vi "RequestInsertSignals.vi"(5 "Events":T1[](array[typedef]), 11 "error in (no error)":errorcluster) -> (6 "request":string, 15 "error out":errorcluster)   [LabVIEW 2019, in "Logger.lvclass"]
uses:
  Logger.lvclass
  SignalData.ctl
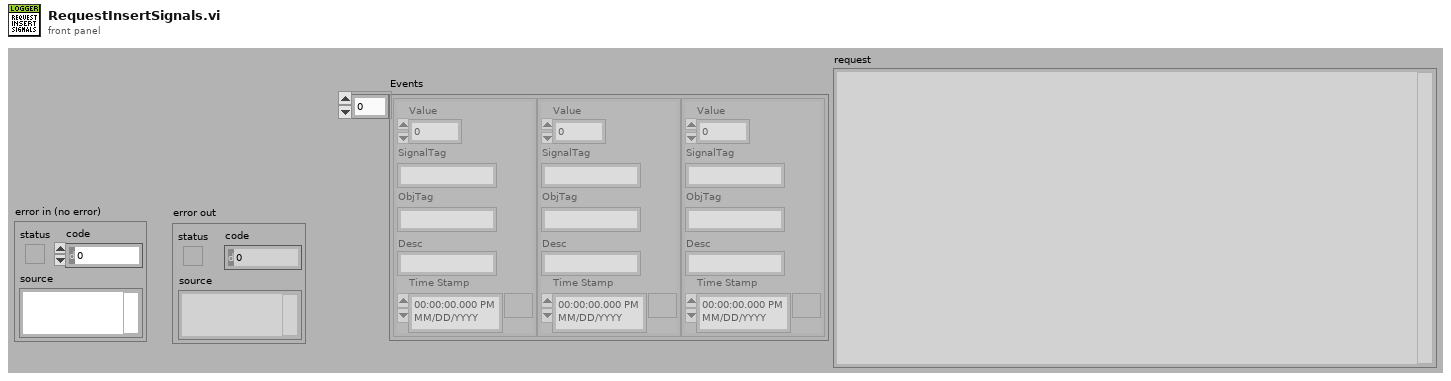
[diagram p1: front panel]
types:
  T1 = typedef "Logger.lvclass/SignalData.ctl" = cluster{"Value":dbl, "SignalTag":string, "ObjTag":string, "Desc":string, "Time Stamp":timestamp}
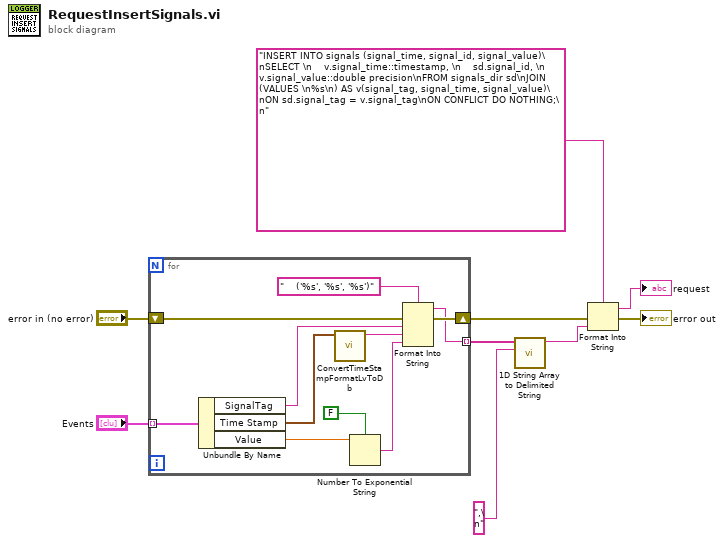
[diagram p0: block diagram]
diagram:
  n1 = for {
    tunnel: [w19] -> w8 mode=indexing
    tunnel: "Events" -> [w16] mode=indexing
    shift-right: [w20] -> w3
    shift-left: "error in (no error)" -> [w18]
    n2 = Unbundle By Name(w16) -> ("SignalTag"=w15:string, "Time Stamp"=w13:timestamp, "Value"=w11:dbl)
    n3 = call "ConvertTimeStampFormatLvToDb.vi"("Time Stamp"=w13) -> ("output string"=w12:string)  [unwired: 10 in]
    n4 = Number To Exponential String(number=w11, 1:FALSE ("use system decimal point (T)")) -> (E-format string=w10:string)  [unwired: 2 in]
    n5 = Format Into String(format string="    ('%s', '%s', '%s')", error in=w18, w15, w12, w10) -> (resulting string=w19:string, error out=w20:errorcluster)  [unwired: 1 in]
  }
  n6 = call <vilib>:"1D String Array to Delimited String.vi"("delimiter"=",\n", "string array"=w8) -> ("delimited string"=w4:string)  [unwired: 9 in]
  n7 = Format Into String(format string="INSERT INTO signals (signal_time, signal_id, signal_value)\nSELECT \n    v.signal_time::timestamp, \n    sd.signal_id, \n    v.signal_value::double precision\nFROM signals_dir sd\nJOIN (VALUES \n%s\n) AS v(signal_tag, signal_time, signal_value)\nON sd.signal_tag = v.signal_tag\nON CONFLICT DO NOTHING;\n", error in=w3, w4) -> (resulting string=→"request":string, error out=→"error out":errorcluster)  [unwired: 1 in]
